vi "brc_daq_get_channels_data.vi"(0 "t0_in":timestamp, 1 "samples_per_ch":i32, 2 "ch_number":i32, 3 "dt":dbl, 5 "error in (no error)":errorcluster, 6 "mHandle":i32, 7 "time_out_ms":i32=5000) -> (14 "t0_out":timestamp, 16 "data_out":waveform(dbl)[](array[waveform]), 19 "error out":errorcluster)   [LabVIEW 2015, in "BRC-DAQ x64.lvlib"]
uses:
  BRC-DAQ x64.lvlib
  DLL/brc_daq_sdk.dll
panel:
  out "size(s)":i32[](array[numeric])
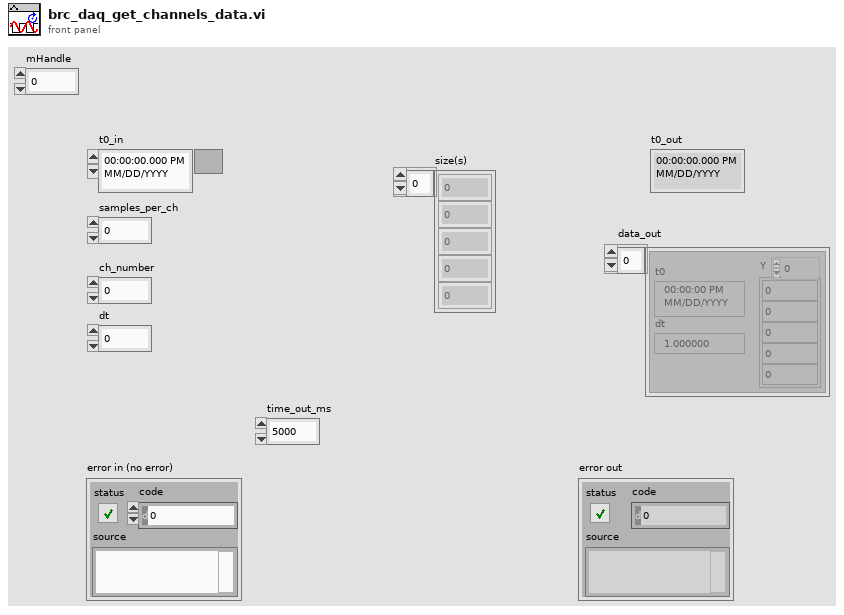
[diagram p1: front panel]
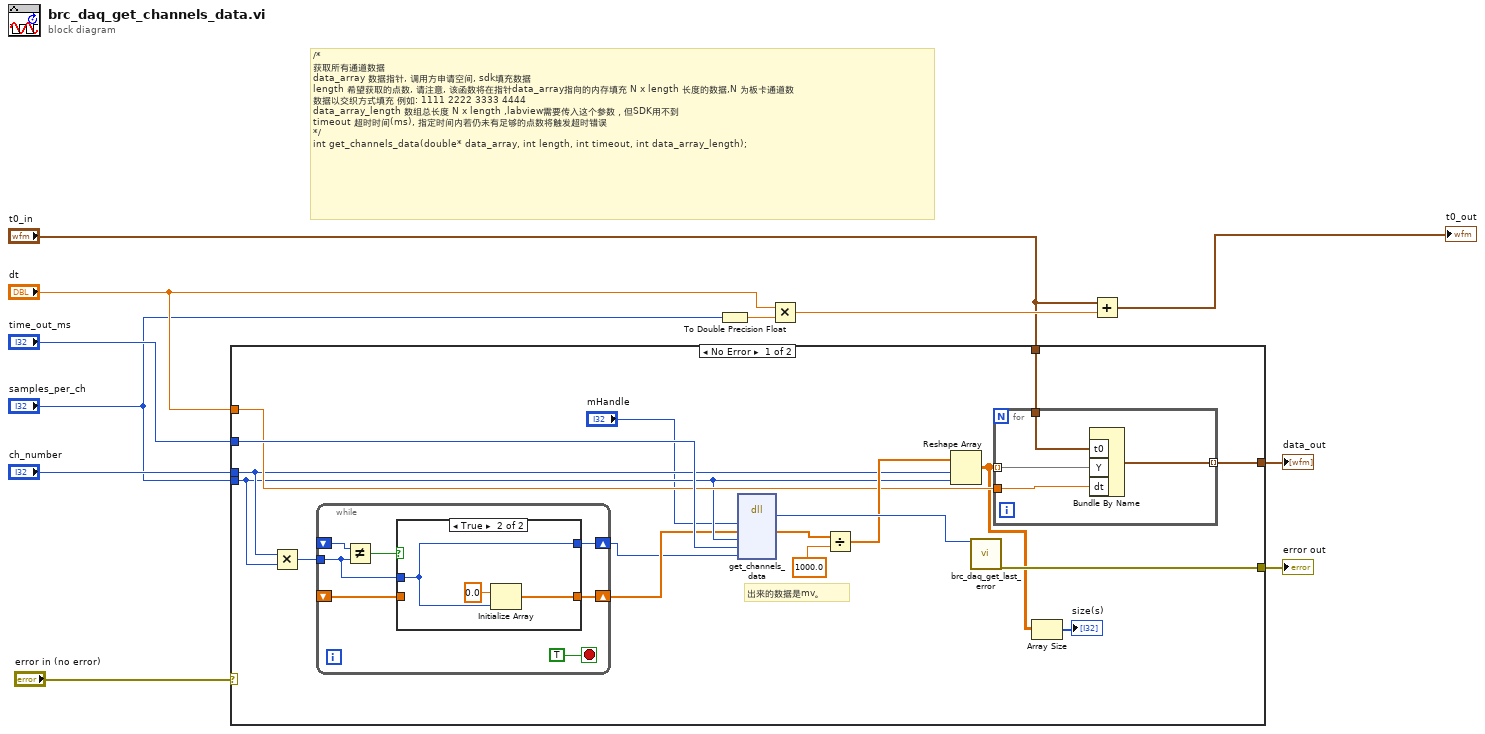
[diagram p0: block diagram]
diagram:
  # "/*\n获取所有通道数据\ndata_array 数据指针, 调用方申请空间, sdk填充数据\nlength 希望获取的点数, 请注意, 该函数将在指针data_array指向的内存填充 N x length 长度的数据,N 为板卡通道数\n数据以交织方式填充 例如: 1111 2222 3333 4444\ndata_array_length 数组总长度 N x length ,labview需要传入这个参数，但SDK用不到\ntimeout 超时时间(ms), 指定时间内若仍未有足够的点数将触发超时错误\n*/\nint get_channels_data(double* data_array, int length, int timeout, int data_array_length);"
  n1 = case shown="No Error" "error in (no error)" {
    selector: "error in (no error)" -> [_ w45]
    tunnel: [w25 w45] -> w11
    tunnel: "time_out_ms" -> [w27 _]
    tunnel: "ch_number" -> [w19 _]
    tunnel: "samples_per_ch" -> [w18 _]
    tunnel: [w28 _] -> w7
    tunnel: "dt" -> [w21 _]
    tunnel: "t0_in" -> [w20 _]
    frame No Error {
      # "出来的数据是mv。"
      n2 = Multiply(x=w19, y=w18) -> (x*y=w17:i32)
      n3 = while {
        shift-right: [w32] -> w15
        shift-left: _ -> [w34]
        tunnel: w17 -> [w31]
        shift-right: [w30] -> w16
        shift-left: _ -> [w29]
        stop <- TRUE stop-if-true
        n4 = Not Equal?(x=w34, y=w31) -> (x != y?=w33:bool)
        n5 = case shown="True" w33 {
          tunnel: [w37 w40] -> w32
          tunnel: w31 -> [w37 w40]
          tunnel: [w36 w38] -> w30
          tunnel: w29 -> [w36 _]
          frame False {
          }
          frame True {
            n6 = Initialize Array(0.0 ("element"), w40) -> (w38:dbl[])
          }
        }
      }
      n7 = dll-call lib="E:/01 BRC project/04BRC-daq/04 Drive/BRC-DAQ/DAQ-x64/DLL/brc_daq_sdk.dll" fn="get_channels_data"("mHandle"="mHandle", "data_array"=w16, "length"=w18, "timeout"=w27, "data_array_length"=w15) -> ("return type"=w26:i32, "data_array"=w24:dbl[])  [unwired: 7 in, 2 out]
      n8 = Divide(x=w24, y=1000.0) -> (x/y=w23:dbl[])
      n9 = Reshape Array(w23, w19, w18) -> (w14:dbl[][])
      n10 = call "brc_daq_get_last_error.vi"("return_value"=w26) -> ("error out"=w25:errorcluster)  [unwired: 18 in]
      n11 = for {
        tunnel: w14 -> [w44] mode=indexing
        tunnel: [w43] -> w28 mode=indexing
        tunnel: w21 -> [w42]
        tunnel: w20 -> [w41]
        n12 = Bundle By Name("t0"=w41, "Y"=w44, "dt"=w42) -> (w43:waveform(dbl))  [unwired: 1 in]
      }
      n13 = Array Size(array=w14) -> (size(s)=→"size(s)":i32[])
    }
    frame Error {
    }
  }
  "error out" <- w11
  "data_out" <- w7
  n14 = To Double Precision Float(number="samples_per_ch") -> (double precision float=w6:dbl)
  n15 = Multiply(x="dt", y=w6) -> (x*y=w5:dbl)
  n16 = Add(x="t0_in", y=w5) -> (x+y=→"t0_out":timestamp)
